vi "MD5 Message Digest.vi"   [LabVIEW 2009]
doc: "Implements the MD5 algorithm to produce a 128-Bit Hash condensed representation of a message or a data file.\n\nPolymorphic VI can output MD5 Hash as Binary String or Hexadeximal String."
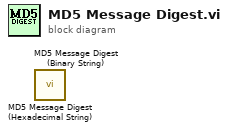
[diagram p0: block diagram]
diagram:
  n1 = call "MD5 Message Digest (Hexadecimal String).vi"() -> ()  [unwired: 1 in, 1 out]
  n2 = call "MD5 Message Digest (Binary String).vi"() -> ()  [unwired: 1 in, 1 out]
